vi "Get Event Id Mapped to Bit Number in Operation Event Register.vi"(8 "error in (no error)":errorcluster, 10 "Bit Number":i32, 11 "VISA resource name":refnum<visa-resource-name>) -> (0 "error out":errorcluster, 1 "Clear Event":i32, 2 "Set Event":i32, 3 "VISA resource name out":refnum<visa-resource-name>)   [LabVIEW 2018, in "Keithley 2450.lvlib"]
doc: "This gets Set Event Id and Clear Event Id Mapped to Bit Number in Operation Event Register."
uses:
  <instrlib>/Keithley 2450/Keithley 2450.lvlib
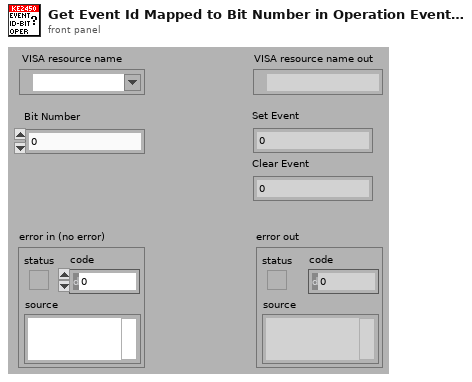
[diagram p1: front panel]
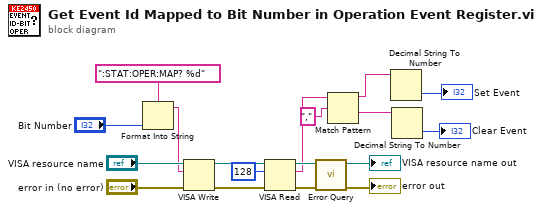
[diagram p0: block diagram]
diagram:
  n1 = Format Into String(format string=":STAT:OPER:MAP? %d", "Bit Number") -> (resulting string=w7:string)  [unwired: 2 in, 1 out]
  n2 = VISA Write(VISA resource name="VISA resource name", write buffer=w7, error in (no error)="error in (no error)") -> (VISA resource name out=w13:refnum<visa-resource-name>, error out=w14:errorcluster)  [unwired: 1 out]
  n3 = VISA Read(VISA resource name=w13, byte count=u32 128, error in (no error)=w14) -> (VISA resource name out=w11:refnum<visa-resource-name>, read buffer=w6:string, error out=w10:errorcluster)  [unwired: 1 out]
  n4 = call <instrlib>:"Error Query.vi"("error in (no error)"=w10, "VISA resource name"=w11) -> ("error out"=→"error out":errorcluster, "VISA resource name out"=→"VISA resource name out":refnum<visa-resource-name>)  [unwired: 8 out]
  n5 = Match Pattern(string=w6, regular expression="," ("search string/char (-)")) -> (before substring=w4:string, after substring=w3:string)  [unwired: 1 in, 2 out]
  n6 = Decimal String To Number(string=w4) -> (number=→"Set Event":i32)  [unwired: 2 in, 1 out]
  n7 = Decimal String To Number(string=w3) -> (number=→"Clear Event":i32)  [unwired: 2 in, 1 out]
